vi "Joystick_Attack3.vi"(11 "JoystickDevRef":T2) -> (3 "Joystick_Attack3":T1)   [LabVIEW 2017]
uses:
  <vilib>/Rock Robotics/WPI/Joystick/WPI_JoystickDevRef.ctl
  <vilib>/Rock Robotics/WPI/Joystick/WPI_JoystickDeviceEnum.ctl
panel:
  out "Generic_Buttons":bool[](array[boolean])
  out "Generic_Axes":dbl[](array[numeric])
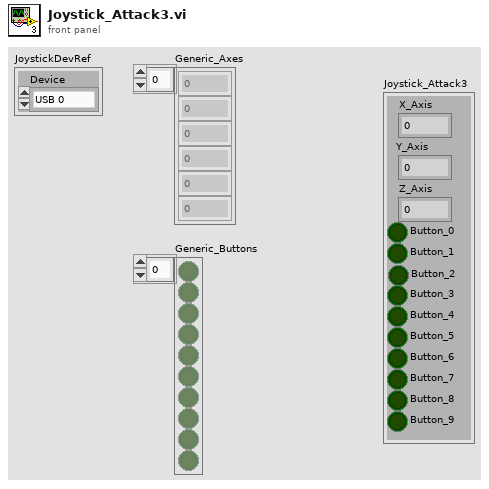
[diagram p1: front panel]
types:
  T1 = cluster{"X_Axis":dbl, "Y_Axis":dbl, "Z_Axis":dbl, "Button_0":bool, "Button_1":bool, "Button_2":bool, "Button_3":bool, "Button_4":bool, "Button_5":bool, "Button_6":bool, "Button_7":bool, "Button_8":bool, "Button_9":bool}
  T2 = typedef "WPI_JoystickDevRef.ctl" = cluster{"Device":T3}
  T3 = typedef "WPI_JoystickDeviceEnum.ctl" = enum16{"USB 0", "USB 1", "USB 2", "USB 3", "USB 4", "USB 5"}
  T4 = cluster{"upper limit":dbl, "upper limit":dbl, "upper limit":dbl, bool, bool, bool, bool, bool, bool, bool, bool, bool, bool}
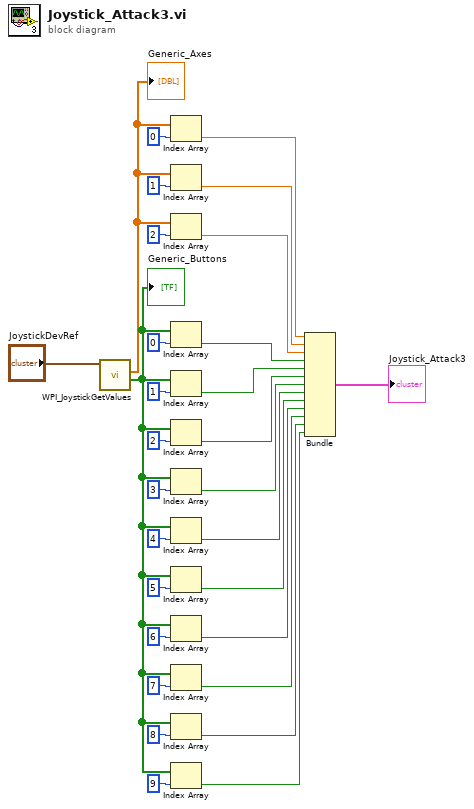
[diagram p0: block diagram]
diagram:
  n1 = call <vilib>:"WPI_JoystickGetValues.vi"("JoystickDevRef"="JoystickDevRef") -> ("Buttons"=w20:bool[], "Axes"=w16:dbl[])  [unwired: 6 in, 3 out]
  "Generic_Axes" <- w16
  "Generic_Buttons" <- w20
  n2 = Index Array(array=w16, index=0) -> (element=w15:dbl)
  n3 = Index Array(array=w16, index=1) -> (element=w14:dbl)
  n4 = Index Array(array=w16, index=2) -> (element=w13:dbl)
  n5 = Index Array(array=w20, index=0) -> (element=w12:bool)
  n6 = Index Array(array=w20, index=1) -> (element=w11:bool)
  n7 = Index Array(array=w20, index=2) -> (element=w10:bool)
  n8 = Index Array(array=w20, index=3) -> (element=w9:bool)
  n9 = Index Array(array=w20, index=4) -> (element=w8:bool)
  n10 = Index Array(array=w20, index=5) -> (element=w7:bool)
  n11 = Index Array(array=w20, index=6) -> (element=w6:bool)
  n12 = Index Array(array=w20, index=7) -> (element=w5:bool)
  n13 = Index Array(array=w20, index=8) -> (element=w4:bool)
  n14 = Index Array(array=w20, index=9) -> (element=w3:bool)
  n15 = Bundle("upper limit"=w15, "upper limit"=w14, "upper limit"=w13, w12, w11, w10, w9, w8, w7, w6, w5, w4, w3) -> (→"Joystick_Attack3":T4)  [unwired: 1 in]
